vi "EvaluateTriggerOpStateExitCondition.vi"(7 "data group":string, 8 "error in":errorcluster, 9 "map":T1, 10 "current op state":i32, 11 "operating states in":variant) -> (0 "error out":errorcluster, 1 "exit":bool, 3 "operating states out":variant)   [LabVIEW 2017, in "OpState.lvlib"]
uses:
  <vilib>/addons/InsightCM/Devices/Shared/Common/OpState/OpState.lvlib
  <vilib>/addons/PointValueMap/controls/PointMap.ctl
  <vilib>/addons/InsightCM/Devices/Shared/Common/OpState/controls/ConditionType.ctl
  <vilib>/addons/InsightCM/Devices/Shared/Common/Trigger/Trigger.lvlib
  <vilib>/addons/PointValueMap/PointValueMap.lvlib
panel:
  out "weight":i32
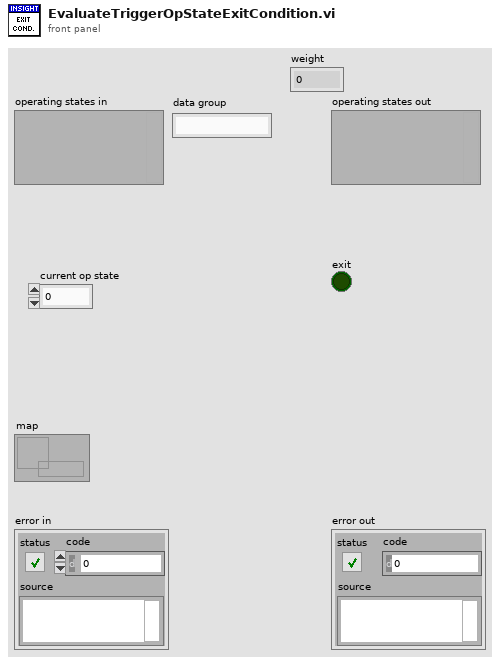
[diagram p1: front panel]
types:
  T1 = typedef "PointValueMap.lvlib/PointMap.ctl" = refnum<data-value>
  T2 = typedef "OpState.lvlib/ConditionType.ctl" = enum16{"Enter", "Exit"}
  T3 = typedef "Trigger.lvlib/TriggerCondition.ctl" = cluster{"Condition":T4, "LatchValue":string, "LatchTime":timestamp}
  T4 = typedef "Condition.ctl" = cluster{"Source":string, "Type":string, "Operator":string, "CompareTo":string, "DwellSeconds":dbl}
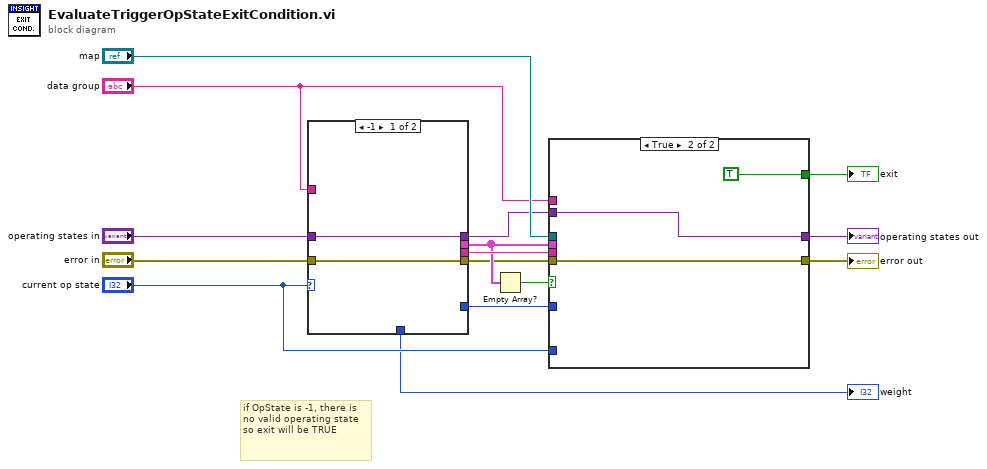
[diagram p0: block diagram]
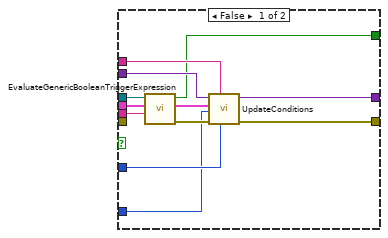
[diagram p2: hidden frame]
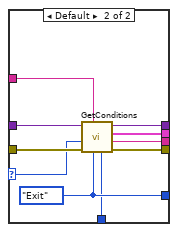
[diagram p3: hidden frame]
diagram:
  # "if OpState is -1, there is no valid operating state so exit will be TRUE"
  n1 = case shown="-1" "current op state" {
    selector: "current op state" -> [_ w24]
    tunnel: "error in" -> [w16 w27]
    tunnel: "operating states in" -> [w17 w26]
    tunnel: "data group" -> [_ w25]
    tunnel: [_ w22] -> w11
    tunnel: [_ w23] -> w10
    tunnel: [w17 w21] -> w8
    tunnel: [w16 w20] -> w7
    tunnel: [_ w19] -> w6
    tunnel: [_ w18] -> w1
    frame -1 {
      # "No Operating State"
    }
    frame Default {
      w19 = ConditionType."Exit" ("ConditionType")
      n2 = call <vilib>:"GetConditions.vi"("condition type"=w19, "data group"=w25, "error in (no error)"=w27, "operating state"=w24, "operating states in"=w26) -> ("error out"=w20:errorcluster, "expression"=w22:string, "conditions"=w23:T3[], "operating states out"=w21:variant, "weight"=w18:i32)  [unwired: 2 in]
    }
  }
  "weight" <- w1
  n3 = Empty Array?(array=w10) -> (empty?=w9:bool)
  n4 = case shown="True" w9 {
    tunnel: [w33 w41] -> w4
    tunnel: "map" -> [w39 _]
    tunnel: [w28 TRUE ("trigger")] -> w5
    tunnel: w11 -> [w38 _]
    tunnel: w10 -> [w37 _]
    tunnel: w8 -> [w35 w42]
    tunnel: [w34 w42] -> w13
    tunnel: w7 -> [_ w41]
    tunnel: w6 -> [w32 _]
    tunnel: "data group" -> [w31 _]
    tunnel: "current op state" -> [w29 _]
    frame False {
      n5 = call <vilib>:"EvaluateGenericBooleanTriggerExpression.vi"("expression"=w38, "all conditions"=w37, "map"=w39) -> ("error out"=w36:errorcluster, "all conditions out"=w30:T3[], "trigger"=w28:bool)  [unwired: 5 in, 1 out]
      n6 = call <vilib>:"UpdateConditions.vi"("ConditionType"=w32, "data group"=w31, "error in (no error)"=w36, "OpState"=w29, "conditions"=w30, "operating states in"=w35) -> ("error out"=w33:errorcluster, "operating states out"=w34:variant)  [unwired: 4 in]
    }
    frame True {
    }
  }
  "error out" <- w4
  "exit" <- w5
  "operating states out" <- w13
